vi "A_star_test.vi"(11 "GIC Input":T1={"     Use ?\nOff       On"=[FALSE, TRUE, FALSE, TRUE], "Mode:"=FALSE, "Extra Port"="", "Hokuyo Port"="COM7", "Tx Prop  Port"="COM6", "Compass Port"="", "GPS Port"="", "Num of WPs"=0, "WP Lats and Longs"={"WP Lats"=[], "WP Longs"=[]}, "Obst Lats and Longs"={"Obst Lats"=[], "Obst Longs"=[]}, "Parameters"=[], "GPS Data"=[], "Compass"=0.0, "LMS Vector"=[], "Vision Vector"=[], "Direction Cmd"=0.0, "Speed Cmd"=0.0, "WP Vector"=[], "WP Number"=0, "Extra"=0, "SW Map"=[], "Path Cluster"={"Path x node"=[], "Path y node"=[]}, "Sim Course"=[]} {"Obst Lats and Longs"."Obst Longs" format="%#_8g"; "Obst Lats and Longs"."Obst Lats" format="%#_8g"}) -> (3 "GIC Output":T1={"     Use ?\nOff       On"=[FALSE, TRUE, FALSE, TRUE], "Mode:"=FALSE, "Extra Port"="", "Hokuyo Port"="COM7", "Tx Prop  Port"="COM6", "Compass Port"="", "GPS Port"="", "Num of WPs"=0, "WP Lats and Longs"={"WP Lats"=[], "WP Longs"=[]}, "Obst Lats and Longs"={"Obst Lats"=[], "Obst Longs"=[]}, "Parameters"=[], "GPS Data"=[], "Compass"=0.0, "LMS Vector"=[], "Vision Vector"=[], "Direction Cmd"=0.0, "Speed Cmd"=0.0, "WP Vector"=[], "WP Number"=0, "Extra"=0, "SW Map"=[], "Path Cluster"={"Path x node"=[], "Path y node"=[]}, "Sim Course"=[]} {"Obst Lats and Longs"."Obst Longs" format="%#_8g"; "Obst Lats and Longs"."Obst Lats" format="%#_8g"})   [LabVIEW 2014]
panel:
  out "map":picture
  in  "Path for GIC":T2
  out "Path":cluster{"Row":dbl, "Col":dbl}[](array[cluster])
  out "sw_map_weights":dbl[][](array[numeric])
  in  "gradient":dbl=10.0
  in  "layers":dbl=3.0
  out "Nodes":cluster{"Weight":dbl, "Row":dbl, "Col":dbl}[][](array[cluster])
  out "Cost_so_far":T3(array[cluster])
  out "Came_from":T4(array[cluster])
  out "Cost So Far":T5
  in  "Goal":cluster{"Weight":dbl, "Row":dbl, "Col":dbl}
  out "Came From":T6
  out "Frontier":cluster{"Weight":dbl, "Row":dbl, "Col":dbl}[](array[cluster])
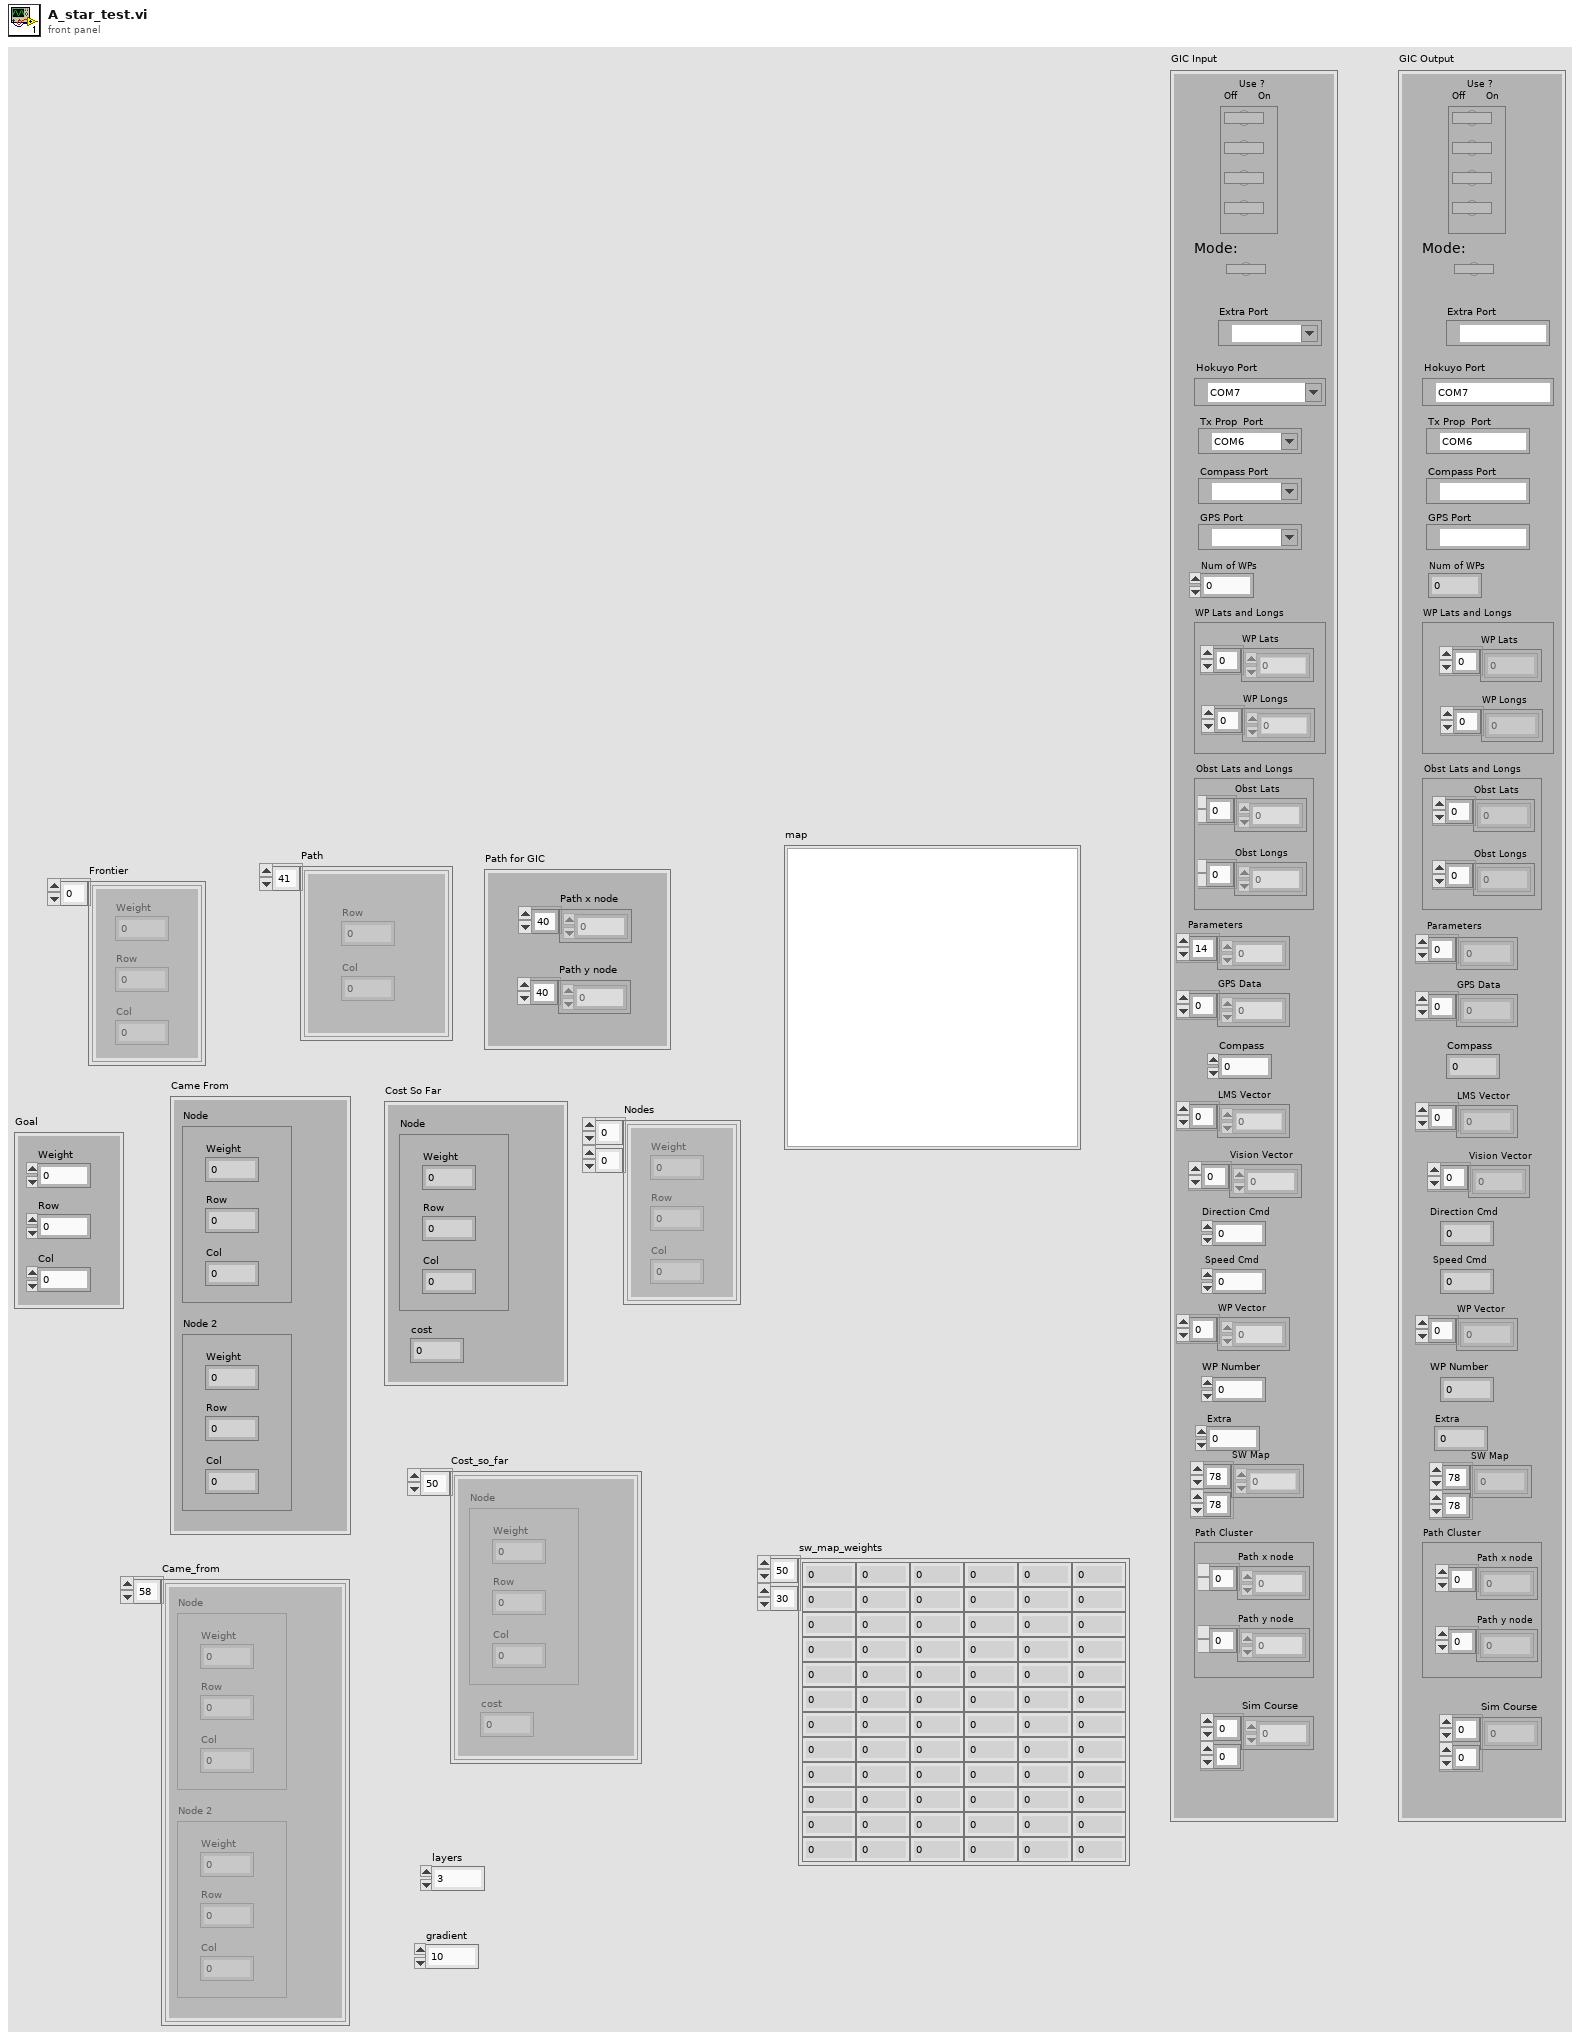
[diagram p1: front panel]
types:
  T1 = cluster{"     Use ?\nOff       On":bool[], "Mode:":bool, "Extra Port":refnum<visa-resource-name>, "Hokuyo Port":refnum<visa-resource-name>, "Tx Prop  Port":refnum<visa-resource-name>, "Compass Port":refnum<visa-resource-name>, "GPS Port":refnum<visa-resource-name>, "Num of WPs":i16, "WP Lats and Longs":cluster{"WP Lats":dbl[], "WP Longs":dbl[]}, "Obst Lats and Longs":cluster{"Obst Lats":dbl[], "Obst Longs":dbl[]}, "Parameters":dbl[], "GPS Data":dbl[], "Compass":dbl, "LMS Vector":dbl[], "Vision Vector":dbl[], "Direction Cmd":dbl, "Speed Cmd":dbl, "WP Vector":dbl[], "WP Number":i32, "Extra":i16, "SW Map":i32[][], "Path Cluster":cluster{"Path x node":dbl[], "Path y node":dbl[]}, "Sim Course":i8[][]}
  T2 = cluster{"Path x node":dbl[], "Path y node":dbl[]}
  T3 = cluster{"Node":cluster{"Weight":dbl, "Row":dbl, "Col":dbl}, "cost":dbl}[]
  T4 = cluster{"Node":cluster{"Weight":dbl, "Row":dbl, "Col":dbl}, "Node 2":cluster{"Weight":dbl, "Row":dbl, "Col":dbl}}[]
  T5 = cluster{"Node":cluster{"Weight":dbl, "Row":dbl, "Col":dbl}, "cost":dbl}
  T6 = cluster{"Node":cluster{"Weight":dbl, "Row":dbl, "Col":dbl}, "Node 2":cluster{"Weight":dbl, "Row":dbl, "Col":dbl}}
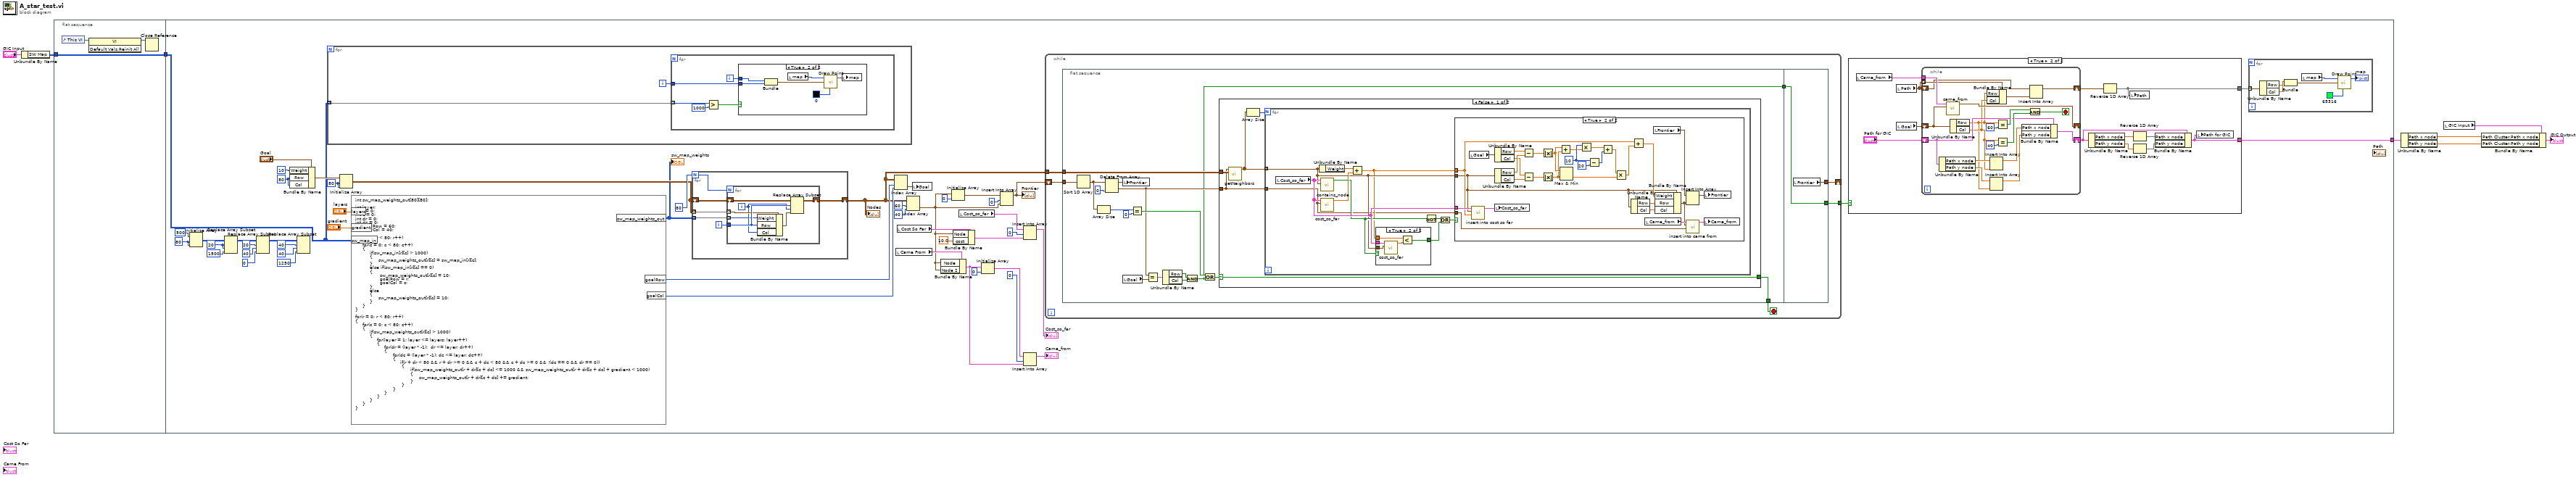
[diagram p0: block diagram]
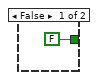
[diagram p5: hidden frame]
diagram:
  n1 = Unbundle By Name("GIC Input") -> ("SW Map"=w8:i32[][])
  n2 = flat-sequence {
    tunnel: w8 -> [w11]
    tunnel: [w11] -> w7
    tunnel: w7 -> [w12]
    tunnel: [w13] -> w6
    frame #0 {
      n3 = control-ref of="This VI"() -> (w10:refnum<vi>)
      n4 = invoke class="VI" method="Default Vals.Reinit All"(reference=w10) -> (reference out=w9:refnum<vi>)  [unwired: 2 in, 2 out]
      n5 = Close Reference(reference=w9) -> ()  [unwired: 1 in, 1 out]
    }
    frame #1 {
      w30 = 20
      w50 = 80
      w56 = 80
      w60 = 80
      n6 = Initialize Array(500, w50, w50) -> (w31:i32[][])
      n7 = Replace Array Subset(array=w31, new element=1500, index (row)=w30, index (col)=w30) -> (w23:i32[][])
      n8 = Replace Array Subset(array=w23, new element=0, index (row)=20, index (col)=40) -> (w17:i32[][])
      n9 = Bundle By Name(cluster="Goal", "Weight"=10, "Row"=w56, "Col"=w56) -> (w55:cluster{"Weight":dbl, "Row":dbl, "Col":dbl})
      n10 = Replace Array Subset(array=w17, new element=1250, index (row)=40, index (col)=40) -> ()  [unwired: 1 out]
      n11 = for {
        tunnel: w12 -> [w70] mode=indexing
        i -> [w69]
        n12 = for {
          tunnel: w70 -> [w75] mode=indexing
          tunnel: w69 -> [w72]
          i -> [w71]
          n13 = Greater?(x=w75, y=1000) -> (0:w73:bool)
          n14 = case shown="True" w73 {
            tunnel: w72 -> [_ w79]
            tunnel: w71 -> [_ w80]
            frame False {
            }
            frame True {
              n15 = Bundle(w80, w79) -> (w78:cluster{i32, i32})  [unwired: 1 in]
              n16 = local read "map"() -> (w77:picture)
              n17 = call <vilib>:"Draw Point.vi"("picture"=w77, "point(x,y)"=w78, "color(black)"=u32 0) -> ("new picture"=w76:picture)  [unwired: 6 in]
              n18 = local write "map"(w76) -> ()
            }
          }
        }
      }
      n19 = Initialize Array(w55, w60, w60) -> (w59:cluster{"Weight":dbl, "Row":dbl, "Col":dbl}[][])
      n20 = formula code="int sw_map_weights_out[80][80];\n\nint layer;\nint r = 0;\nint c = 0;\nint dr = 0;\nint dc = 0;\nint goalRow = 60;\nint goalCol = 40;\n\nfor(r = 0; r < 80; r++)\n{\n     for(c = 0; c < 80; c++)\n     {\n          if(sw_map_in[r][c] > 1000)\n          {\n                sw_map_weights_out[r][c] = sw_map_in[r][c];\n          }\n          else if(sw_map_in[r][c] == 0)\n          {\n                 sw_map_weights_out[r][c] = 10;\n                 goalRow = r;\n                 goalCol = c;\n          }\n          else\n          {\n                sw_map_weights_out[r][c] = 10;\n          }\n     }\n}\n\nfor(r = 0; r < 80; r++)\n{\n     for(c = 0; c < 80; c++)\n     {\n          if(sw_map_weights_out[r][c] > 1000)\n          {\n               for(layer = 1; layer <= layers; layer++)\n               {\n                    for(dr = (layer * -1);  dr <= layer; dr++)\n                    {\n                          for(dc = (layer * -1); dc <= layer; dc++)\n                          {\n                               if(r + dr < 80 && r + dr >= 0 && c + dc < 80 && c + dc >= 0 && !(dc == 0 && dr == 0))\n                                {\n                                      if(sw_map_weights_out[r + dr][c + dc] <= 1000 && sw_map_weights_out[r + dr][c + dc] + gradient < 1000)\n                                      {\n                                            sw_map_weights_out[r + dr][c + dc] += gradient;\n                                      }\n                                }\n                          }\n                    }\n               }\n          }\n     }\n}"("layers"="layers", "gradient"="gradient", "sw_map_in"=w12) -> ("sw_map_weights_out"=w28:i32[][], "goalRow"=w27:i32, "goalCol"=w26:i32)
      "sw_map_weights" <- w28
      n21 = for {
        N: 80 -> [w114]
        tunnel: w59 -> [w119] mode=indexing
        shift-right: [w116] -> w24
        shift-left: w59 -> [w118]
        tunnel: w28 -> [w115] mode=indexing
        i -> [w117]
        n22 = for {
          N: w114 -> [_]
          tunnel: w119 -> [w124] mode=indexing
          tunnel: w117 -> [w125]
          shift-right: [w122] -> w116
          shift-left: w118 -> [w126]
          tunnel: w115 -> [w121] mode=indexing
          i -> [w123]
          n23 = Bundle By Name(cluster=w124, "Weight"=w121, "Row"=w125, "Col"=w123) -> (w120:cluster{"Weight":dbl, "Row":dbl, "Col":dbl})
          n24 = Replace Array Subset(array=w126, new element=w120, index (row)=w125, index (col)=w123) -> (w122:cluster{"Weight":dbl, "Row":dbl, "Col":dbl}[][])
        }
      }
      "Nodes" <- w24
      n25 = Index Array(array=w24, index (row)=w27, index (col)=w26) -> (element=w25:cluster{"Weight":dbl, "Row":dbl, "Col":dbl})
      n26 = local read "Came From"() -> (w45:T6)
      n27 = local read "Cost So Far"() -> (w40:T5)
      n28 = Index Array(array=w24, index (row)=60, index (col)=40) -> (element=w39:cluster{"Weight":dbl, "Row":dbl, "Col":dbl})
      n29 = local write "Goal"(w25) -> ()
      n30 = Bundle By Name(cluster=w45, "Node"=w39, "Node 2"=w39) -> (w42:T6)
      n31 = Initialize Array(w39, 0) -> (w48:cluster{"Weight":dbl, "Row":dbl, "Col":dbl}[])
      n32 = Bundle By Name(cluster=w40, "Node"=w39, "cost"=10.0) -> (w37:T5)
      n33 = local read "Cost_so_far"() -> (w36:T3)
      n34 = Initialize Array(w42, 0) -> (w44:T4)
      n35 = Insert Into Array(array=w48, index=0, new element=w39) -> (w47:cluster{"Weight":dbl, "Row":dbl, "Col":dbl}[])
      "Frontier" <- w47
      n36 = Insert Into Array(array=w36, index=0, new element=w37) -> (→"Cost_so_far":T3)
      n37 = Insert Into Array(array=w44, index=0, new element=w42) -> (→"Came_from":T4)
      n38 = while {
        tunnel: w24 -> [w131]
        shift-right: [w129] -> _
        shift-left: w47 -> [w132]
        tunnel: [w127] -> w19
        stop <- w130 stop-if-true
        n39 = flat-sequence {
          tunnel: w132 -> [w146]
          tunnel: w131 -> [w141]
          tunnel: [w139] -> w130
          tunnel: [w133] -> w128
          tunnel: [w202] -> w129
          tunnel: w128 -> [w201]
          tunnel: [w201] -> w127
          frame #0 {
            n40 = Sort 1D Array(array=w146) -> (sorted array=w145:cluster{"Weight":dbl, "Row":dbl, "Col":dbl}[])
            n41 = Array Size(array=w145) -> (size(s)=w147:i32)
            n42 = Delete From Array(array=w145, index=0) -> (deleted portion=w140:cluster{"Weight":dbl, "Row":dbl, "Col":dbl}, array with subset deleted=w138:cluster{"Weight":dbl, "Row":dbl, "Col":dbl}[])  [unwired: 1 in]
            n43 = local write "Frontier"(w138) -> ()
            n44 = local read "Goal"() -> (w142:cluster{"Weight":dbl, "Row":dbl, "Col":dbl})
            n45 = Equal?(x=w147, y=0) -> (x = y?=w143:bool)
            n46 = Equal?(x=w140, y=w142) -> (x = y?=w137:cluster{"Weight":bool, "Row":bool, "Col":bool})
            n47 = Unbundle By Name(w137) -> ("Row"=w136:bool, "Col"=w135:bool)
            n48 = And(x=w136, y=w135) -> (x .and. y?=w133:bool)
            n49 = Or(x=w143, y=w133) -> (x .or. y?=w134:bool)
            n50 = case shown="False" w134 {
              selector: w134 -> [w152 w200]
              tunnel: w141 -> [w153 _]
              tunnel: w140 -> [w151 _]
              tunnel: [w152 w200] -> w139
              frame False {
                n51 = call "getNeighbors.vi"("Nodes"=w153, "Node"=w151) -> ("neighbors"=w150:cluster{"Weight":dbl, "Row":dbl, "Col":dbl}[])  [unwired: 9 in]
                n52 = Array Size(array=w150) -> (size(s)=w149:i32)
                n53 = for {
                  N: w149 -> [_]
                  tunnel: w150 -> [w156] mode=indexing
                  tunnel: w151 -> [w154]
                  n54 = local read "Cost_so_far"() -> (w158:T3)
                  n55 = Unbundle By Name(w156) -> ("Weight"=w162:dbl)
                  n56 = call "contains_node.vi"("Node"=w156, "Cost_so_far"=w158) -> ("output"=w157:bool)  [unwired: 9 in]
                  n57 = call "cost_so_far.vi"("Node"=w154, "Cost_so_far"=w158) -> ("cost out"=w163:dbl)  [unwired: 9 in]
                  n58 = Add(x=w162, y=w163) -> (x+y=w155:dbl)
                  n59 = case shown="True" w157 {
                    tunnel: w155 -> [_ w197]
                    tunnel: w158 -> [_ w199]
                    tunnel: w156 -> [_ w198]
                    tunnel: [FALSE w195] -> w160
                    frame False {
                    }
                    frame True {
                      n60 = call "cost_so_far.vi"("Node"=w198, "Cost_so_far"=w199) -> ("cost out"=w196:dbl)  [unwired: 9 in]
                      n61 = Less?(x=w197, y=w196) -> (x < y?=w195:bool)
                    }
                  }
                  n62 = Not(x=w157) -> (.not. x?=w161:bool)
                  n63 = Or(x=w161, y=w160) -> (x .or. y?=w159:bool)
                  n64 = case shown="True" w159 {
                    tunnel: w158 -> [_ w193]
                    tunnel: w156 -> [_ w180]
                    tunnel: w155 -> [_ w192]
                    tunnel: w154 -> [_ w185]
                    frame False {
                    }
                    frame True {
                      w172 = 10
                      n65 = local read "Goal"() -> (w181:cluster{"Weight":dbl, "Row":dbl, "Col":dbl})
                      n66 = call "insert into cost so far.vi"("new cost"=w192, "Node"=w180, "Cost_so_far"=w193) -> ("cost_so_far output"=w183:T3)  [unwired: 8 in]
                      n67 = Unbundle By Name(w181) -> ("Row"=w179:dbl, "Col"=w175:dbl)
                      n68 = Unbundle By Name(w180) -> ("Row"=w178:dbl, "Col"=w174:dbl)
                      n69 = local write "Cost_so_far"(w183) -> ()
                      n70 = Subtract(x=w179, y=w178) -> (x-y=w177:dbl)
                      n71 = Subtract(x=w175, y=w174) -> (x-y=w176:dbl)
                      n72 = Absolute Value(x=w177) -> (abs(x)=w167:dbl)
                      n73 = Absolute Value(x=w176) -> (abs(x)=w166:dbl)
                      n74 = Add(x=w167, y=w166) -> (x+y=w171:dbl)
                      n75 = Max & Min(x=w167, y=w166) -> (min(x,y)=w165:dbl)  [unwired: 1 out]
                      n76 = Multiply(x=w172, y=w171) -> (x*y=w170:dbl)
                      n77 = Subtract(x=w172, y=20) -> (x-y=w169:i32)
                      n78 = Add(x=w170, y=w169) -> (x+y=w168:dbl)
                      n79 = Multiply(x=w168, y=w165) -> (x*y=w164:dbl)
                      n80 = Unbundle By Name(w180) -> ("Row"=w190:dbl, "Col"=w189:dbl)
                      n81 = Add(x=w192, y=w164) -> (x+y=w191:dbl)
                      n82 = local read "Came_from"() -> (w187:T4)
                      n83 = local read "Frontier"() -> (w188:cluster{"Weight":dbl, "Row":dbl, "Col":dbl}[])
                      n84 = Bundle By Name(cluster=w180, "Weight"=w191, "Row"=w190, "Col"=w189) -> (w186:cluster{"Weight":dbl, "Row":dbl, "Col":dbl})
                      n85 = Insert Into Array(array=w188, new element=w186) -> (w182:cluster{"Weight":dbl, "Row":dbl, "Col":dbl}[])  [unwired: 1 in]
                      n86 = call "insert into came from.vi"("Node came from"=w185, "Node"=w186, "Came_from"=w187) -> ("Came_from out"=w184:T4)  [unwired: 8 in]
                      n87 = local write "Frontier"(w182) -> ()
                      n88 = local write "Came_from"(w184) -> ()
                    }
                  }
                }
              }
              frame True {
              }
            }
          }
          frame #1 {
            n89 = local read "Frontier"() -> (w202:cluster{"Weight":dbl, "Row":dbl, "Col":dbl}[])
          }
        }
      }
      n90 = case shown="True" w19 {
        tunnel: [_ w83] -> w18
        tunnel: [_ w82] -> w13
        frame False {
        }
        frame True {
          n91 = local read "Came_from"() -> (w93:T4)
          n92 = local read "Path"() -> (w91:cluster{"Row":dbl, "Col":dbl}[])
          n93 = local read "Goal"() -> (w92:cluster{"Weight":dbl, "Row":dbl, "Col":dbl})
          n94 = while {
            shift-right: [w106] -> _
            shift-left: w92 -> [w108]
            tunnel: w93 -> [w107]
            tunnel: w91 -> [w105] mode=indexing
            shift-right: [w102] -> w90
            shift-left: w91 -> [w104]
            shift-right: [w96] -> w86
            shift-left: "Path for GIC" -> [w99]
            stop <- w109 stop-if-true
            n95 = Unbundle By Name(w99) -> ("Path x node"=w101:dbl[], "Path y node"=w100:dbl[])
            n96 = call "came_from.vi"("Node"=w108, "Came_from"=w107) -> ("Node came from"=w106:cluster{"Weight":dbl, "Row":dbl, "Col":dbl})  [unwired: 9 in]
            n97 = Unbundle By Name(w108) -> ("Row"=w94:dbl, "Col"=w95:dbl)
            n98 = Bundle By Name(cluster=w105, "Row"=w94, "Col"=w95) -> (w103:cluster{"Row":dbl, "Col":dbl})
            n99 = Insert Into Array(array=w101, new element=w95) -> (w97:dbl[])  [unwired: 1 in]
            n100 = Insert Into Array(array=w100, new element=w94) -> (w98:dbl[])  [unwired: 1 in]
            n101 = Equal?(x=w94, y=60) -> (x = y?=w111:bool)
            n102 = Equal?(x=w95, y=40) -> (x = y?=w110:bool)
            n103 = Bundle By Name(cluster=w99, "Path x node"=w97, "Path y node"=w98) -> (w96:T2)
            n104 = And(x=w111, y=w110) -> (x .and. y?=w109:bool)
            n105 = Insert Into Array(array=w104, new element=w103) -> (w102:cluster{"Row":dbl, "Col":dbl}[])  [unwired: 1 in]
          }
          n106 = Unbundle By Name(w86) -> ("Path x node"=w88:dbl[], "Path y node"=w87:dbl[])
          n107 = Reverse 1D Array(array=w90) -> (reversed array=w83:cluster{"Row":dbl, "Col":dbl}[])
          n108 = local write "Path"(w83) -> ()
          n109 = Reverse 1D Array(array=w88) -> (reversed array=w85:dbl[])
          n110 = Reverse 1D Array(array=w87) -> (reversed array=w84:dbl[])
          n111 = Bundle By Name(cluster=w86, "Path x node"=w85, "Path y node"=w84) -> (w82:T2)
          n112 = local write "Path for GIC"(w82) -> ()
        }
      }
      n113 = for {
        tunnel: w18 -> [w67] mode=indexing
        n114 = Unbundle By Name(w67) -> ("Row"=w65:dbl, "Col"=w66:dbl)
        n115 = Bundle("Col"=w66, "Row"=w65) -> (w64:cluster{"Col":dbl, "Row":dbl})  [unwired: 1 in]
        n116 = local read "map"() -> (w68:picture)
        n117 = call <vilib>:"Draw Point.vi"("picture"=w68, "point(x,y)"=w64, "color(black)"=u32 65316) -> ("new picture"=→"map":picture)  [unwired: 6 in]
      }
    }
  }
  n118 = Unbundle By Name(w6) -> ("Path x node"=w5:dbl[], "Path y node"=w4:dbl[])
  n119 = local read "GIC Input"() -> (w2:T1)
  n120 = Bundle By Name(cluster=w2, "Path Cluster.Path x node"=w5, "Path Cluster.Path y node"=w4) -> (→"GIC Output":T1)
